vi "CC Generate Script Text.vi"(8 "error in (no error)":errorcluster, 11 "Script":T1[](array[typedef])) -> (0 "error out":errorcluster, 3 "Script String":string)   [LabVIEW 2024]
uses:
  typedefs/CC Script Step.ctl
  typedefs/CC enum Script Action.ctl
  typedefs/CC cluster Object.ctl
  typedefs/CC cluster sidereal rate.ctl
  typedefs/CC cluster RA and DEC.ctl
  typedefs/cc cluster muRA muDEC.ctl
  Telescope/CC cluster Telescope Offsets.ctl
  typedefs/CC cluster Exposure.ctl
  Detector/Detector Class/Detector enum Detector Integration Mode.ctl
  typedefs/CC Dithering.ctl
  typedefs/CC cluster Offset Dithering.ctl
  typedefs/CC Dithering Offsets.ctl
  typedefs/CC cluster Random Dithering.ctl
  typedefs/CC cluster Acquire Parameters.ctl
  typedefs/CC cluster Filter Wheel Parameters.ctl
  Focus/Focus cluster MoveFocus Command Parameters.ctl
  typedefs/CC cluster Pause Parameters.ctl
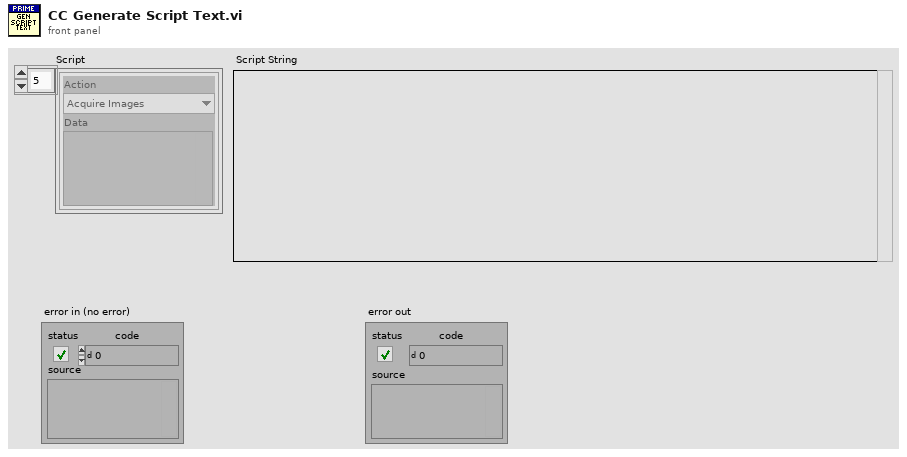
[diagram p1: front panel]
types:
  T1 = typedef "CC Script Step.ctl" = cluster{"Action":T2, "Data":variant}
  T2 = typedef "CC enum Script Action.ctl" = enum16{"Noop", "Define Object", "Define Exposure", "Define Dithering", "Acquire Images", "Set Filter Wheel", "Telescope Home", "Telescope Move", "Telescope RA DEC", "Focus Move Relative", "Focus Move Absolute", "Focus Set Home", "Macro", "Pause", "Ask User", "Define Random Dither"}
  T3 = typedef "CC cluster Object.ctl" = cluster{"Object":cluster{"Name":string}, "Sidereal Rate":T4, "RA and DEC":T5, "muRA muDEC Epoch":T6, "Offsets":T7}
  T4 = typedef "CC cluster sidereal rate.ctl" = cluster{"dRA":dbl, "dDEC":dbl}
  T5 = typedef "CC cluster RA and DEC.ctl" = cluster{"RA":dbl, "DEC":dbl}
  T6 = typedef "cc cluster muRA muDEC.ctl" = cluster{"muRA":dbl, "muDEC":dbl, "Epoch":dbl}
  T7 = typedef "CC cluster Telescope Offsets.ctl" = cluster{"RA":dbl, "DEC":dbl, "ROT":dbl}
  T8 = typedef "CC cluster Exposure.ctl" = cluster{"Mode":T9, "Integration Time":dbl, "Name":string, "Images":i32}
  T9 = typedef "Detector enum Detector Integration Mode.ctl" = enum16{"SSR", "CDS", "MEAN", "MEDIAN", "MODE", "MIIN", "MAX"}
  T10 = typedef "CC Dithering.ctl" = cluster{"Name":string, "Dithering Offsets":T11}
  T11 = typedef "CC cluster Offset Dithering.ctl" = cluster{"Offsets":T12[]}
  T12 = typedef "CC Dithering Offsets.ctl" = cluster{"DEC":dbl, "RA":dbl}
  T13 = typedef "CC cluster Random Dithering.ctl" = cluster{"Count":i32, "Radius":dbl, "Name":string}
  T14 = typedef "CC cluster Acquire Parameters.ctl" = cluster{"Object":string, "Exposure":string, "Dithering":string}
  T15 = typedef "CC cluster Filter Wheel Parameters.ctl" = cluster{"Wheel":i32, "Filter":i32}
  T16 = typedef "Focus cluster MoveFocus Command Parameters.ctl" = cluster{"Motor":i32, "Position":i32}
  T17 = typedef "CC cluster Pause Parameters.ctl" = cluster{"Time (s)":dbl}
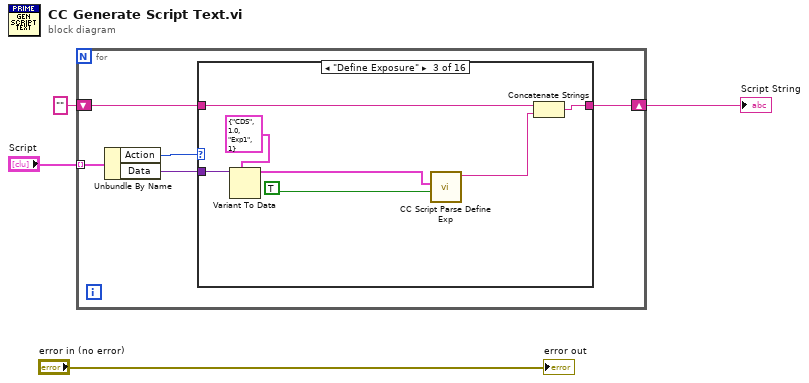
[diagram p0: block diagram]
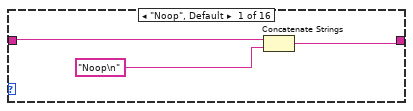
[diagram p2: hidden frame]
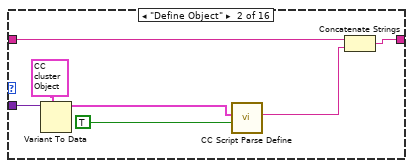
[diagram p3: hidden frame]
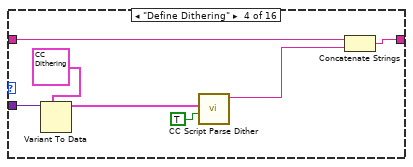
[diagram p4: hidden frame]
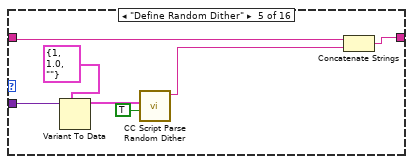
[diagram p5: hidden frame]
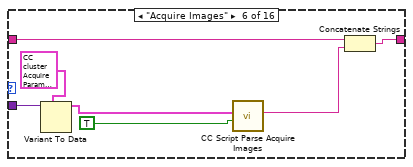
[diagram p6: hidden frame]
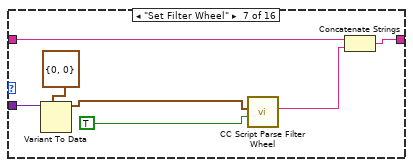
[diagram p7: hidden frame]
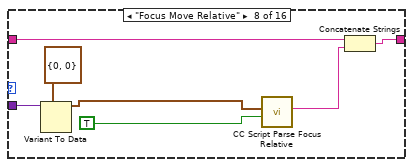
[diagram p8: hidden frame]
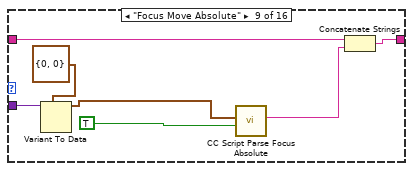
[diagram p9: hidden frame]
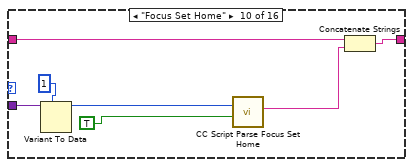
[diagram p10: hidden frame]
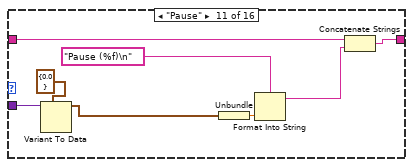
[diagram p11: hidden frame]
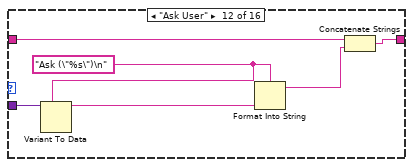
[diagram p12: hidden frame]
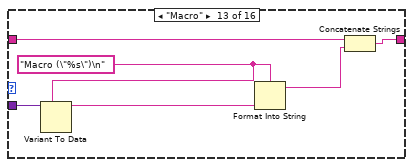
[diagram p13: hidden frame]
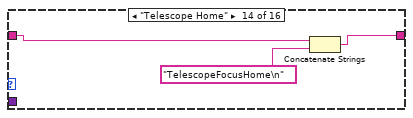
[diagram p14: hidden frame]
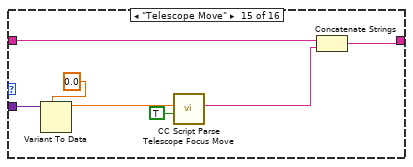
[diagram p15: hidden frame]
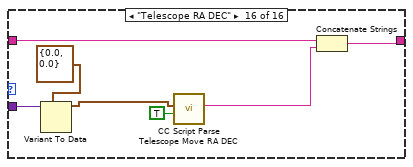
[diagram p16: hidden frame]
diagram:
  n1 = for {
    tunnel: "Script" -> [w9] mode=indexing
    shift-right: [w6] -> w1
    shift-left: "" -> [w5]
    n2 = Unbundle By Name(w9) -> ("Action"=w8:T2, "Data"=w7:variant)
    n3 = case shown="\"Define Exposure\"" w8 {
      tunnel: w7 -> [_ w19 w26 w33 w39 w47 w54 w61 w68 w75 w83 w89 w95 _ w105 w112]
      tunnel: [w11 w14 w25 w32 w36 w46 w53 w60 w67 w74 w82 w88 w94 w97 w99 w108] -> w6
      tunnel: w5 -> [w12 w13 w24 w31 w35 w45 w52 w59 w66 w73 w81 w87 w93 w98 w101 w110]
      frame "Noop", Default {
        n4 = Concatenate Strings(w12, "Noop\n" ("string")) -> (w11:string)
      }
      frame "Define Object" {
        n5 = Variant To Data(type=T3 {"Object"={"Name"=""}, "Sidereal Rate"={"dRA"=0.0, "dDEC"=0.0}, "RA and DEC"={"RA"=0.0, "DEC"=0.0}, "muRA muDEC Epoch"={"muRA"=0.0, "muDEC"=0.0, "Epoch"=0.0}, "Offsets"={"RA"=0.0, "DEC"=0.0, "ROT"=0.0}} ("Object"), Variant=w19) -> (data=w17:T3)  [unwired: 1 in, 1 out]
        n6 = call "CC Script Parse Define.vi"("To String?"=TRUE, "Object in"=w17) -> ("Script"=w15:string)  [unwired: 6 in, 3 out]
        n7 = Concatenate Strings(w13, w15) -> (w14:string)
      }
      frame "Define Exposure" {
        n8 = Variant To Data(type=T8 {"Mode"=enum."CDS", "Integration Time"=1.0, "Name"="Exp1", "Images"=1} ("Exposure in"), Variant=w26) -> (data=w22:T8)  [unwired: 1 in, 1 out]
        n9 = call "CC Script Parse Define Exp.vi"("To String?"=TRUE, "Exposure in"=w22) -> ("Script String out"=w20:string)  [unwired: 6 in, 3 out]
        n10 = Concatenate Strings(w24, w20) -> (w25:string)
      }
      frame "Define Dithering" {
        n11 = Variant To Data(type=T10 {"Name"="", "Dithering Offsets"={"Offsets"=[{"DEC"=0.0, "RA"=0.0}, {"DEC"=-10.0, "RA"=-10.0}]}} ("Dithering Offsets in"), Variant=w33) -> (data=w29:T10)  [unwired: 1 in, 1 out]
        n12 = call "CC Script Parse Dither.vi"("To String?"=TRUE, "Dithering in"=w29) -> ("resulting string"=w28:string)  [unwired: 7 in, 2 out]
        n13 = Concatenate Strings(w31, w28) -> (w32:string)
      }
      frame "Define Random Dither" {
        n14 = Variant To Data(type=T13 {"Count"=1, "Radius"=1.0, "Name"=""} ("Dithering Offsets in"), Variant=w39) -> (data=w38:T13)  [unwired: 1 in, 1 out]
        n15 = call "CC Script Parse Random Dither.vi"("To String?"=TRUE, "Dithering in"=w38) -> ("resulting string"=w34:string)  [unwired: 7 in, 2 out]
        n16 = Concatenate Strings(w35, w34) -> (w36:string)
      }
      frame "Acquire Images" {
        n17 = Variant To Data(type=T14 {"Object"="Alpha1234", "Exposure"="Exp1", "Dithering"="Dither2"} ("Acquire Parameters in"), Variant=w47) -> (data=w43:T14)  [unwired: 1 in, 1 out]
        n18 = call "CC Script Parse Acquire Images.vi"("To Script?"=TRUE ("To String?"), "Acquire Parameters in"=w43) -> ("Script out"=w41:string)  [unwired: 7 in, 2 out]
        n19 = Concatenate Strings(w45, w41) -> (w46:string)
      }
      frame "Set Filter Wheel" {
        n20 = Variant To Data(type=T15 {"Wheel"=0, "Filter"=0} ("Acquire Parameters in"), Variant=w54) -> (data=w50:T15)  [unwired: 1 in, 1 out]
        n21 = call "CC Script Parse Filter Wheel.vi"("To Script?"=TRUE ("To String?"), "Filter Wheel parameters in"=w50) -> ("Script Out"=w48:string)  [unwired: 7 in, 2 out]
        n22 = Concatenate Strings(w52, w48) -> (w53:string)
      }
      frame "Focus Move Relative" {
        n23 = Variant To Data(type=T16 {"Motor"=0, "Position"=0} ("Cluster"), Variant=w61) -> (data=w58:T16)  [unwired: 1 in, 1 out]
        n24 = call "CC Script Parse Focus Relative.vi"("To Script?"=TRUE ("To String?"), "Move parm in"=w58) -> ("Script Out"=w56:string)  [unwired: 7 in, 2 out]
        n25 = Concatenate Strings(w59, w56) -> (w60:string)
      }
      frame "Focus Move Absolute" {
        n26 = Variant To Data(type=T16 {"Motor"=0, "Position"=0} ("Cluster"), Variant=w68) -> (data=w65:T16)  [unwired: 1 in, 1 out]
        n27 = call "CC Script Parse Focus Absolute.vi"("To Script?"=TRUE ("To String?"), "Move parm in"=w65) -> ("Script Out"=w63:string)  [unwired: 7 in, 2 out]
        n28 = Concatenate Strings(w66, w63) -> (w67:string)
      }
      frame "Focus Set Home" {
        n29 = Variant To Data(type=1 ("Set Home parm in"), Variant=w75) -> (data=w71:i32)  [unwired: 1 in, 1 out]
        n30 = call "CC Script Parse Focus Set Home.vi"("To Script?"=TRUE ("To String?"), "Set Home parm in"=w71) -> ("Script Out"=w69:string)  [unwired: 7 in, 2 out]
        n31 = Concatenate Strings(w73, w69) -> (w74:string)
      }
      frame "Pause" {
        n32 = Variant To Data(type=T17 {"Time (s)"=0.0} ("Acquire Parameters in"), Variant=w83) -> (data=w78:T17)  [unwired: 1 in, 1 out]
        n33 = Unbundle(w78) -> ("Time (s)"=w77:dbl)
        n34 = Format Into String(format string="Pause (%f)\n", w77) -> (resulting string=w76:string)  [unwired: 2 in, 1 out]
        n35 = Concatenate Strings(w81, w76) -> (w82:string)
      }
      frame "Ask User" {
        w85 = "Ask (\"%s\")\n" ("format string")
        n36 = Variant To Data(type=w85, Variant=w89) -> (data=w84:string)  [unwired: 1 in, 1 out]
        n37 = Format Into String(format string=w85, w84) -> (resulting string=w86:string)  [unwired: 2 in, 1 out]
        n38 = Concatenate Strings(w87, w86) -> (w88:string)
      }
      frame "Macro" {
        w91 = "Macro (\"%s\")\n" ("format string")
        n39 = Variant To Data(type=w91, Variant=w95) -> (data=w90:string)  [unwired: 1 in, 1 out]
        n40 = Format Into String(format string=w91, w90) -> (resulting string=w92:string)  [unwired: 2 in, 1 out]
        n41 = Concatenate Strings(w93, w92) -> (w94:string)
      }
      frame "Telescope Home" {
        n42 = Concatenate Strings(w98, "TelescopeFocusHome\n" ("string")) -> (w97:string)
      }
      frame "Telescope Move" {
        n43 = Variant To Data(type=0.0 ("Focus Move Pos"), Variant=w105) -> (data=w103:dbl)  [unwired: 1 in, 1 out]
        n44 = call "CC Script Parse Telescope Focus Move.vi"("To Script?"=TRUE, "Telescope Move Pos"=w103) -> ("Script Out"=w100:string)  [unwired: 7 in, 2 out]
        n45 = Concatenate Strings(w101, w100) -> (w99:string)
      }
      frame "Telescope RA DEC" {
        n46 = Variant To Data(type=T5 {"RA"=0.0, "DEC"=0.0} ("RA and DEC"), Variant=w112) -> (data=w106:T5)  [unwired: 1 in, 1 out]
        n47 = call "CC Script Parse Telescope Move RA DEC.vi"("To Script?"=TRUE, "RA and DEC"=w106) -> ("Script Out"=w109:string)  [unwired: 7 in, 2 out]
        n48 = Concatenate Strings(w110, w109) -> (w108:string)
      }
    }
  }
  "Script String" <- w1
  "error out" <- "error in (no error)"
